vi "Recurse.vi"(6 "Error":errorcluster, 7 "Actor":refnum<class "Actor.lvclass">, 11 "Msg":refnum<class "Msg.lvclass">) -> (3 "Msg":refnum<class "Msg.lvclass">, 4 "Error":errorcluster, 5 "Actor":refnum<class "Actor.lvclass">)   [LabVIEW 2020, in "_Template.lvlib" / "{{Msg}}.lvlib"]
uses:
  {{Msg}}.lvlib
  Msg/Msg.lvclass
  C:/Users/nathan.davis/Desktop/personal/jettl-harness/repos/jettl/src/jettl Tools/_Template/{{Msg}}/Message/Msg.lvclass
  C:/Users/nathan.davis/Desktop/personal/jettl-harness/repos/jettl/src/jettl/jettl/Message/Message.lvclass
  jettl/jettl/Actor/Actor.lvclass
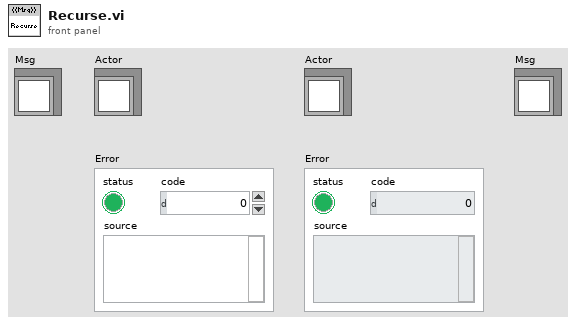
[diagram p1: front panel]
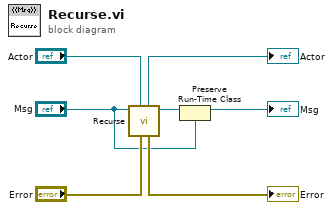
[diagram p0: block diagram]
diagram:
  n1 = call-dynamic "Recurse.vi"("Error"="Error", "Actor"="Actor", "Message"="Msg") -> ("Message"=w5:refnum<class "Message.lvclass">, "Error"=→"Error":errorcluster, "Actor"=→"Actor":refnum<class "Actor.lvclass">)  [unwired: 6 in]
  n2 = Preserve Run-Time Class(object in=w5, 2:"Msg") -> (object out=→"Msg":refnum<class "Msg.lvclass">)  [unwired: 1 in, 1 out]
